vi "Shutdown.vi"(8 "error in":errorcluster, 11 "tCRD in":refnum<class "Aircraft OPCCRD.lvclass">) -> (0 "error out":errorcluster, 3 "tCRD out":refnum<class "Aircraft OPCCRD.lvclass">)   [LabVIEW 2015, in "Aircraft OPCCRD.lvclass"]
uses:
  Aircraft OPCCRD.lvclass
  Aircraft OPCCRD.lvclass/Aircraft OPCCRD.ctl
  Reusable/Observer/Observer.lvclass/Observer.ctl
  <vilib>/FPGAPlugInAG/sbRIO-9636/niLvFpga_Close_sbRIO-9636.vi
  Reusable/CRDS/Main/CRDS.lvclass
  Reusable/Data/Data.lvclass
  <vilib>/rvi/interface/nirviCloseFPGA/nirviCloseFPGA.xnode
  tFPGA Ref.ctl
  FPGA Bitfiles/Aircraft OPCRD Server.lvbitx
  Reusable/Observer/Data Subject.lvclass
  Reusable/Observer/Observer.lvclass
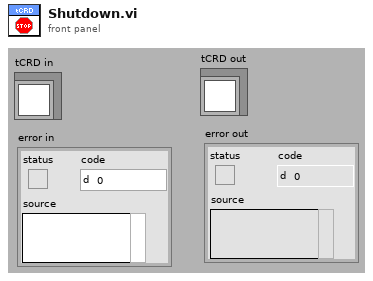
[diagram p1: front panel]
types:
  T1 = typedef "Aircraft OPCCRD.lvclass/tFPGA Ref.ctl" = refnum<k20>
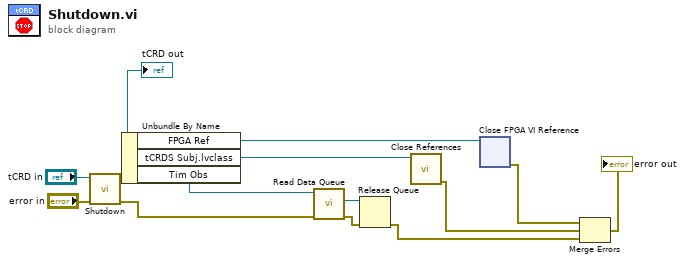
[diagram p0: block diagram]
diagram:
  n1 = call-parent "Shutdown.vi"("error in"="error in", "Instrument in"="tCRD in") -> ("error out"=w8:errorcluster, "Instrument out"=w11:refnum<class "Aircraft OPCCRD.lvclass">)  [unwired: 8 in]
  "tCRD out" <- w11
  n2 = Unbundle By Name(w11) -> ("FPGA Ref"=w10:T1, "tCRDS Subj.lvclass"=w6:refnum<class "tCRDS Subj.lvclass">, "Tim Obs"=w5:refnum<class "Tim File Observer.lvclass">)
  n3 = call "Read Data Queue.vi"("error in (no error)"=w8, "Observer in"=w5) -> ("error out"=w7:errorcluster, "Data Queue"=w9:refnum<queue>)  [unwired: 7 in, 1 out]
  n4 = Release Queue(queue=w9, error in (no error)=w7) -> (error out=w2:errorcluster)  [unwired: 1 in, 2 out]
  n5 = call "Close References.vi"("Data Subject in"=w6) -> ("error out"=w3:errorcluster)  [unwired: 9 in, 1 out]
  n6 = xnode "Close FPGA VI Reference"("FPGA VI Reference In"=w10) -> ("error out"=w4:errorcluster)  [unwired: 1 in]
  n7 = Merge Errors(w4, w3, w2) -> (→"error out":errorcluster)
